vi "Get Data.vi"(8 "error in (no error)":errorcluster, 11 "Message Data in":refnum<class "Message Data.lvclass">) -> (0 "error out":errorcluster, 3 "Message Data out":refnum<class "Message Data.lvclass">)   [LabVIEW 2023, in "Message Data.lvclass"]
uses:
  Message Data.lvclass
  Message Data.lvclass/Message Data.ctl
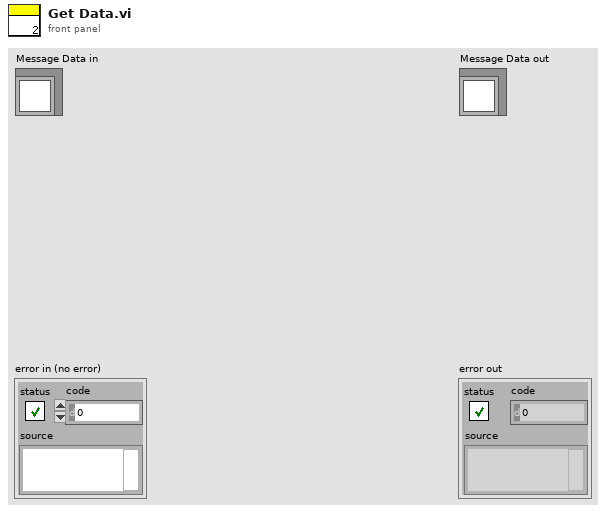
[diagram p1: front panel]
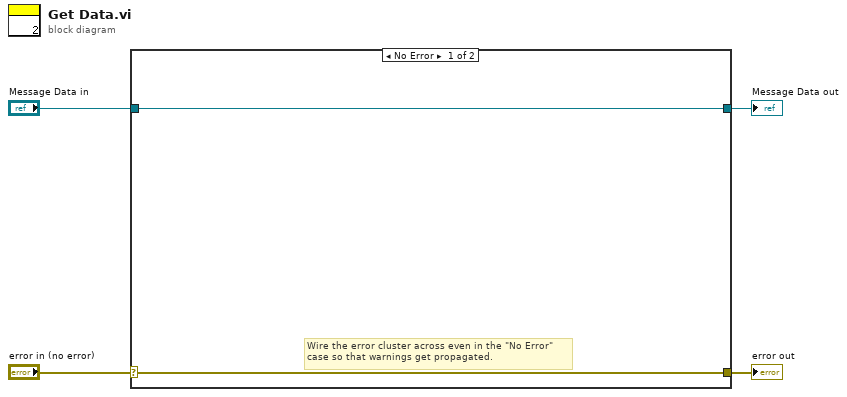
[diagram p0: block diagram]
diagram:
  n1 = case shown="No Error" "error in (no error)" {
    selector: "error in (no error)" -> [w5 w8]
    tunnel: [w5 w8] -> w3
    tunnel: [w6 w7] -> w1
    tunnel: "Message Data in" -> [w6 w7]
    frame No Error {
      # "Wire the error cluster across even in the \"No Error\"\ncase so that warnings get propagated."
    }
    frame Error {
    }
  }
  "error out" <- w3
  "Message Data out" <- w1
